vi "Set - Reset.vi"(1 "Reset":bool, 2 "Set":bool) -> (0 "Output":bool)   [LabVIEW 2015]
doc: "This VI accepts a \"set\" boolean input which when true, sets the value of the output to true and a reset button which when true sets the value of the output to false. In all other cases, nothing happens to he output."
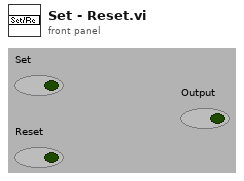
[diagram p1: front panel]
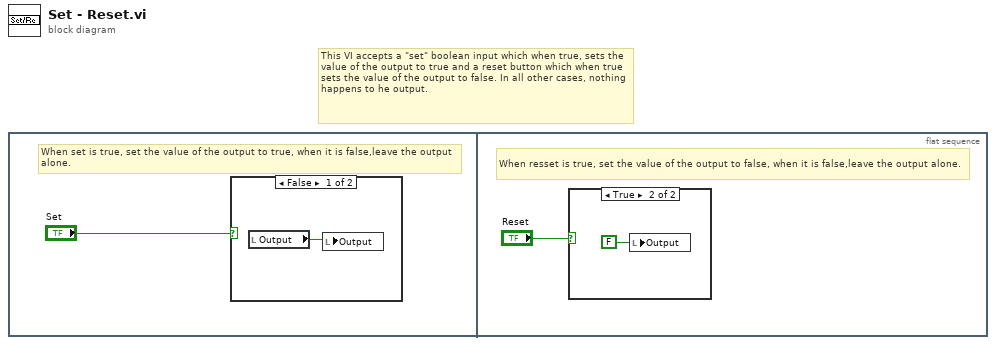
[diagram p0: block diagram]
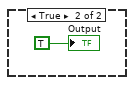
[diagram p2: hidden frame]
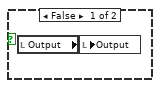
[diagram p3: hidden frame]
diagram:
  # "This VI accepts a \"set\" boolean input which when true, sets the value of the output to true and a reset button which when true sets the value of the output to false. In all other cases, nothing happens to he output."
  n1 = flat-sequence {
    frame #0 {
      # "When set is true, set the value of the output to true, when it is false,leave the output alone."
      n2 = case shown="False" "Set" {
        frame False {
          n3 = local read "Output"() -> (w2:bool)
          n4 = local write "Output"(w2) -> ()
        }
        frame True {
          "Output" <- TRUE ("Output")
        }
      }
    }
    frame #1 {
      # "When resset is true, set the value of the output to false, when it is false,leave the output alone."
      n5 = case shown="True" "Reset" {
        frame False {
          n6 = local read "Output"() -> (w5:bool)
          n7 = local write "Output"(w5) -> ()
        }
        frame True {
          n8 = local write "Output"(FALSE ("Output")) -> ()
        }
      }
    }
  }
